vi "PickeringBlank.vi"(3 "Xmit Ring":i8=1) -> (0 "error out":errorcluster, 2 "dup VISA resource name":refnum<visa-resource-name>)   [LabVIEW 2022 SP3]
panel:
  # "A zero clears all switches. 1-5 selects Xmit ring"
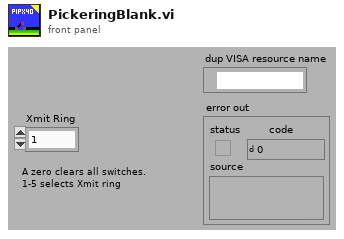
[diagram p1: front panel]
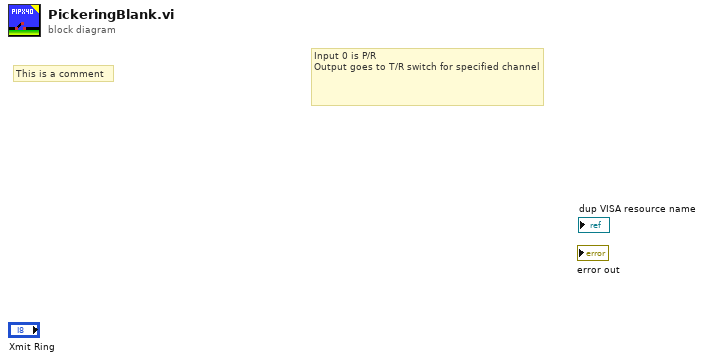
[diagram p0: block diagram]
diagram:
  # "This is a comment"
  # "Input 0 is P/R\nOutput goes to T/R switch for specified channel"
